vi "Light intensity final sub.vi"(8 "error in (no error)":errorcluster, 11 "LINX Resource":T1) -> (2 "Voltage":dbl, 3 "Numeric":i32)   [LabVIEW 2020]
uses:
  <vilib>/MakerHub/LINX/Private/Type Defs/LINX Ref.ctl
  <vilib>/MakerHub/LINX/Private/Type Defs/Platform.ctl
  <vilib>/MakerHub/LINX/Private/Type Defs/Interface.ctl
  <vilib>/MakerHub/LINX/Private/Device/Type Defs/LINX Device Config.ctl
  <vilib>/MakerHub/LINX/Private/Device/Type Defs/TCP Config.ctl
  <vilib>/MakerHub/LINX/Private/Device/Type Defs/Channels.ctl
  <vilib>/MakerHub/LINX/Public/Peripherals/Analog/Analog Read 1 Chan.vi
  <vilib>/MakerHub/LINX/Public/Peripherals/Analog/Analog Read N Chans.vi
  <vilib>/MakerHub/LINX/Private/Local IO/LinxAnalogRead.vi
  <vilib>/MakerHub/LINX/Public/Utilities/Check Channel.vi
  <vilib>/MakerHub/LINX/Private/Utilties/Generate Error.vi
  <vilib>/MakerHub/LINX/LMH-LINX.lvlib
  <vilib>/MakerHub/LINX/Private/Device/Device.lvlib
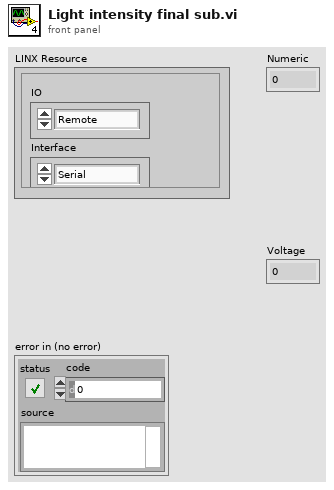
[diagram p1: front panel]
types:
  T1 = typedef "LMH-LINX.lvlib/LINX Ref.ctl" = cluster{"IO":T2, "Interface":T3, "LINX Device Config":T4}
  T2 = typedef "LMH-LINX.lvlib/Platform.ctl" = enum16{"Remote", "Local"}
  T3 = typedef "LMH-LINX.lvlib/Interface.ctl" = enum16{"Serial", "TCP"}
  T4 = typedef "LMH-LINX.lvlib/Device.lvlib/LINX Device Config.ctl" = cluster{"Interface":T3, "COM Port":refnum<visa-resource-name>, "TCP Configuration":T5, "Device Family":u8, "Device ID":u8, "Device Name":string, "TCP Ref":refnum<k5>, "Channels":T6}
  T5 = typedef "LMH-LINX.lvlib/Device.lvlib/TCP Config.ctl" = cluster{"IP Address":string, "Port":u16}
  T6 = typedef "LMH-LINX.lvlib/Channels.ctl" = cluster{"DI":u8[], "DO":u8[], "AI":u8[], "AO":u8[], "PWM":u8[], "QE":u8[], "UART":u8[], "I2C 2":u8[], "SPI":u8[], "CAN":u8[], "Servo":u8[], "AI Ref (V)":dbl, "AI Resolution (Bits)":u8, "AO Ref (V)":dbl, "AO Resolution (Bits)":u8}
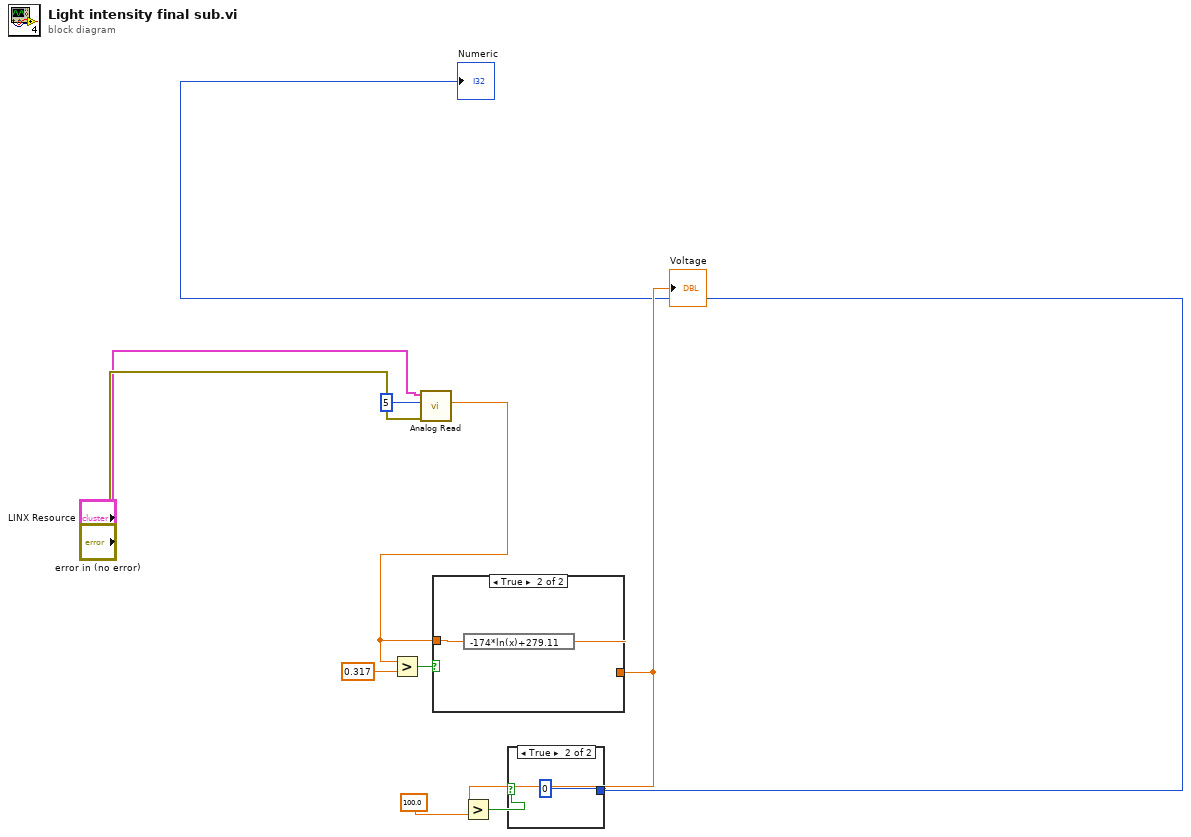
[diagram p0: block diagram]
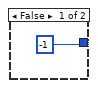
[diagram p2: hidden frame]
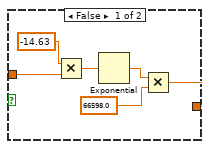
[diagram p3: hidden frame]
diagram:
  n1 = call-poly <vilib>:"Analog Read.vi"("Error In"="error in (no error)", "Analog Channel"=u8 5, "LINX Resource"="LINX Resource") -> ("Voltage"=w5:dbl)  [unwired: 5 in, 3 out]
  n2 = Greater?(x=w5, y=0.317) -> (0:w10:bool)
  n3 = case shown="True" w10 {
    tunnel: w5 -> [w12 w17]
    tunnel: [w13 w18] -> w6
    frame False {
      n4 = Multiply(x=-14.63, y=w12) -> (x*y=w14:dbl)
      n5 = Exponential(1:w14) -> (0:w16:dbl)
      n6 = Multiply(x=w16, y=66598.0) -> (x*y=w13:dbl)
    }
    frame True {
      n7 = expression code="-174*ln(x)+279.11"(w17) -> (w18:dbl)
    }
  }
  "Voltage" <- w6
  n8 = Greater?(x=w6, y=100.0) -> (0:w8:bool)
  n9 = case shown="True" w8 {
    tunnel: [-1 0] -> w1
    frame False {
    }
    frame True {
    }
  }
  "Numeric" <- w1
